vi "init and update listboxes.vi"(8 "error in (no error)":errorcluster, 9 "table":refnum<vi>, 10 "display":refnum<vi>) -> (0 "error out":errorcluster, 2 "selected values":bool[](array[boolean]))   [LabVIEW 2016, in "FPGA Resource Manager.lvlib"]
uses:
  FPGA Resource Manager.lvlib
  global constants.vi
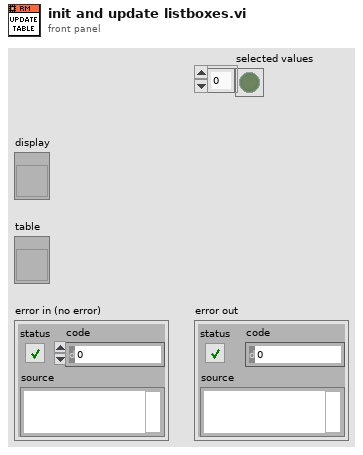
[diagram p1: front panel]
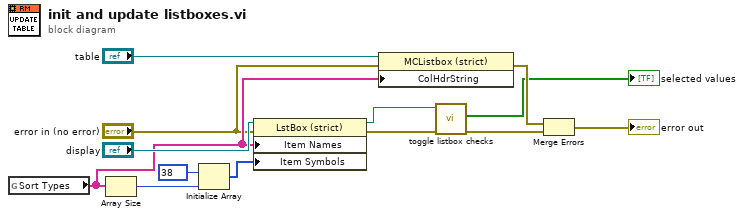
[diagram p0: block diagram]
diagram:
  n1 = global read "global constants.vi" "Sort Types"() -> (w7:string[])
  n2 = Array Size(array=w7) -> (size(s)=w9:i32)
  n3 = Initialize Array(38, w9) -> (w8:i32[])
  n4 = property on="Property Node" class="LstBox (strict)"(reference="display", error in="error in (no error)", "Item Names"=w7, "Item Symbols"=w8) -> (reference out=w12:refnum<vi>, error out=w13:errorcluster)
  n5 = property class="MCListbox (strict)"(reference="table", error in="error in (no error)", "ColHdrString"=w7) -> (error out=w3:errorcluster)  [unwired: 1 out]
  n6 = call "toggle listbox checks.vi"("error in (no error)"=w13, "ListBox in"=w12) -> ("error out"=w5:errorcluster, "selected values"=→"selected values":bool[])  [unwired: 8 in]
  n7 = Merge Errors(w3, w5) -> (→"error out":errorcluster)
